vi "Process Command.vi"(4 "error in (no error)":errorcluster, 7 "Read Graph Data in":refnum<class "Remote Access Commands_Read Graph Data.lvclass">) -> (0 "error out":errorcluster, 2 "Response out":T1, 3 "Read Graph Data out":refnum<class "Remote Access Commands_Read Graph Data.lvclass">)   [LabVIEW 2020, in "Startup Processes.lvlib" / "Remote Access Commands_Read Graph Data.lvclass"]
uses:
  Remote Access Commands_Read Graph Data.lvclass
  Remote Access Commands_Read Graph Data.lvclass/Remote Access Commands_Read Graph Data.ctl
  toolbox/Standard Signalling/not_Generic Named Notifier/not_Generic Named Notifier.lvlib
  _ude/Read Graph Data/Read Graph Data.lvlib
  Remote Access Commands.lvclass
  Startup Processes.lvlib
  _typedefs/Custom Remote Access Error Codes.ctl
  _typedefs/JSON Response Cluster.ctl
  C:/Users/Fred Guo/Desktop/Release 19/_libraries/Startup Processes/_classes/Remote Access Commands/Remote Access Commands.lvclass
  C:/Users/Fred Guo/Desktop/Release 19/_libraries/Startup Processes/_classes/Remote Access Commands/Read Graph Data/Remote Access Commands_Read Graph Data.lvclass
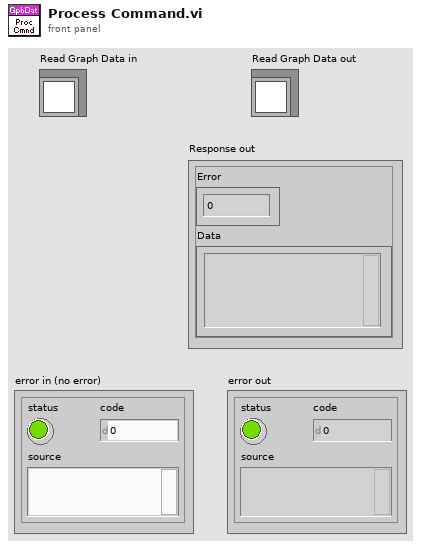
[diagram p1: front panel]
types:
  T1 = typedef "Startup Processes.lvlib/JSON Response Cluster.ctl" = cluster{"Error":i32, "Data":string}
  T2 = typedef "Startup Processes.lvlib/Custom Remote Access Error Codes.ctl" = enum16{"No Error", "CRC Error", "Update Failed"}
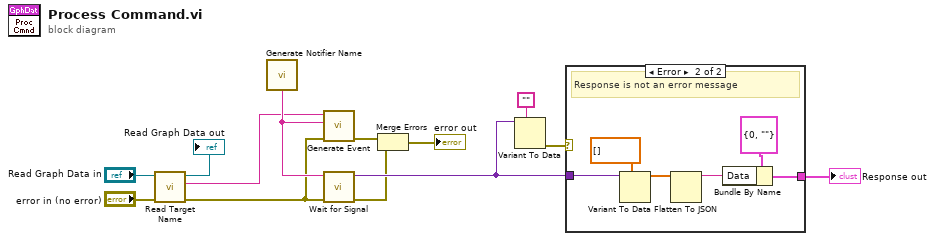
[diagram p0: block diagram]
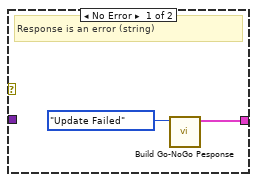
[diagram p2: hidden frame]
diagram:
  n1 = call "Read Target Name.vi"("Error In"="error in (no error)", "Remote Access Commands in"="Read Graph Data in") -> ("Error Out"=w8:errorcluster, "Target Name"=w7:string, "Remote Access Commands out"=→"Read Graph Data out":refnum<class "Remote Access Commands_Read Graph Data.lvclass">)  [unwired: 3 in]
  n2 = call "Generate Notifier Name.vi"() -> ("Notifier Name"=w12:string)
  n3 = call "Generate Event.vi"("Error In"=w8, "Response Notifier"=w12, "Graph Name"=w7) -> ("Error Out"=w13:errorcluster)  [unwired: 4 in]
  n4 = call "Wait for Signal.vi"("Error In"=w8, "Notifier Name"=w12) -> ("Error Out"=w1:errorcluster, "Signal Data"=w5:variant)  [unwired: 4 in]
  n5 = Merge Errors(w13, w1) -> (→"error out":errorcluster)
  n6 = Variant To Data(type="", Variant=w5) -> (error out=w3:errorcluster)  [unwired: 1 in, 1 out]
  n7 = case shown="Error" w3 {
    tunnel: w5 -> [_ w20]
    tunnel: [w14 w16] -> w2
    frame No Error {
      # "Response is an error (string)"
      n8 = call "Build Go-NoGo Pesponse.vi"("Error"=Custom_Remote_Access_Error_Codes."Update Failed") -> ("Response"=w14:T1)  [unwired: 5 in, 1 out]
    }
    frame Error {
      # "Response is not an error message"
      n9 = Variant To Data(type=dbl[] [] ("Waveform Graph"), Variant=w20) -> (data=w19:dbl[])  [unwired: 1 in, 1 out]
      n10 = Flatten To JSON(anything=w19) -> (JSON string=w18:string)  [unwired: 2 in, 1 out]
      n11 = Bundle By Name(cluster=T1 {"Error"=0, "Data"=""} ("Response"), "Data"=w18) -> (w16:T1)
    }
  }
  "Response out" <- w2
